vi "rsidr_core_global.vi"() -> ()   [LabVIEW 2015, in "Rohde&Schwarz CMXP NR FR2 Measurement.lvlib"]
doc: "This Global variable contains driver's:\n- Attributes\n- Range Tables\n- Repeated Capabilities"
uses:
  <instrlib>/Rohde&Schwarz CMXP NR FR2 Measurement/Rohde&Schwarz CMXP NR FR2 Measurement.lvlib
panel:
  out "Attributes":T1(array[cluster])=[{"Level"=1, "Class Only"=TRUE, "Identifier"="", "Descriptive Name"="Configuration", "Data Type"=enum."ViInt32", "Command"="", "Access"=enum."Read Only", "Range Table"="", "Read Callback"="", "Write Callback"="", "Range Callback"="", "Check Callback"="", "Rngtable Callback"="", "Coerce Callback"="", "Supported Models"="", "Instrument Options"="", "Check Status Callback"="", "Flags"=0, "Help"="Configures the NR FR 2 measurement subsystem."}, {"Level"=2, "Class Only"=FALSE, "Identifier"="RSCMXPNRFR2M_ATTR_CONNECTOR", "Descriptive Name"="Connector", "Data Type"=enum."ViInt32", "Command"="ROUT:NRMM:MEAS{instance}:SPAT", "Access"=enum."Read/Write", "Range Table"="rsCmxpNrFr2M_rngInputConnector", "Read Callback"="", "Write Callback"="", "Range Callback"="", "Check Callback"="", "Rngtable Callback"="", "Coerce Callback"="", "Supported Models"="", "Instrument Options"="", "Check Status Callback"="", "Flags"=0, "Help"="Selects the input connector for the measured signal.\n\nAvailable Repeated Capabilities:\ninstance: i0, i1, i2, i3, i4, i5, i6, i7, i8, i9, i10, i11, i12, i13, i14, i15, i16, i17, i18, i19, i20, i21, i22, i23, i24, i25, i26, i27, i28, i29, i30, i31, i32\r\n\nRemote-control command(s):\nROUTe:NRMMw:MEAS<i>:SPATh"}, {"Level"=2, "Class Only"=FALSE, "Identifier"="RSCMXPNRFR2M_ATTR_EXTERNAL_ATTENUATION", "Descriptive Name"="External Attenuation", "Data Type"=enum."ViReal64", "Command"="CONF:NRMM:MEAS{instance}:RFS:EATT", "Access"=enum."Read/Write", "Range Table"="rsCmxpNrFr2M_rngExtAtt", "Read Callback"="", "Write Callback"="", "Range Callback"="", "Check Callback"="", "Rngtable Callback"="", "Coerce Callback"="", "Supported Models"="", "Instrument Options"="", "Check Status Callback"="", "Flags"=0, "Help"="Defines an external attenuation (or gain, if the value is negative), to be applied to the input connector.\n\nAvailable Repeated Capabilities:\ninstance: i0, i1, i2, i3, i4, i5, i6, i7, i8, i9, i10, i11, i12, i13, i14, i15, i16, i17, i18, i19, i20, i21, i22, i23, i24, i25, i26, i27, i28, i29, i30, i31, i32\r\n\nRemote-control command(s):\nCONFigure:NRMMw:MEAS<i>:RFSettings:EATTenuation"}, {"Level"=2, "Class Only"=FALSE, "Identifier"="RSCMXPNRFR2M_ATTR_BAND", "Descriptive Name"="Band", "Data Type"=enum."ViInt32", "Command"="CONF:NRMM:MEAS{instance}:BAND", "Access"=enum."Read/Write", "Range Table"="rsCmxpNrFr2M_rngInputSignalFrequencyBand", "Read Callback"="", "Write Callback"="", "Range Callback"="", "Check Callback"="", "Rngtable Callback"="", "Coerce Callback"="", "Supported Models"="", "Instrument Options"="", "Check Status Callback"="", "Flags"=0, "Help"="Selects the frequency band.\n\nAvailable Repeated Capabilities:\ninstance: i0, i1, i2, i3, i4, i5, i6, i7, i8, i9, i10, i11, i12, i13, i14, i15, i16, i17, i18, i19, i20, i21, i22, i23, i24, i25, i26, i27, i28, i29, i30, i31, i32\r\n\nRemote-control command(s):\nCONFigure:NRMMw:MEAS<i>:BAND"}, {"Level"=2, "Class Only"=FALSE, "Identifier"="RSCMXPNRFR2M_ATTR_FREQUENCY", "Descriptive Name"="Frequency", "Data Type"=enum."ViReal64", "Command"="CONF:NRMM:MEAS{instance}:RFS:FREQ", "Access"=enum."Read/Write", "Range Table"="", "Read Callback"="", "Write Callback"="", "Range Callback"="", "Check Callback"="", "Rngtable Callback"="", "Coerce Callback"="", "Supported Models"="", "Instrument Options"="", "Check Status Callback"="", "Flags"=0, "Help"="Selects the center frequency of the measured carrier.\n\nAvailable Repeated Capabilities:\ninstance: i0, i1, i2, i3, i4, i5, i6, i7, i8, i9, i10, i11, i12, i13, i14, i15, i16, i17, i18, i19, i20, i21, i22, i23, i24, i25, i26, i27, i28, i29, i30, i31, i32\r\n\nRemote-control command(s):\nCONFigure:NRMMw:MEAS<i>:RFSettings:FREQuency"}, {"Level"=2, "Class Only"=FALSE, "Identifier"="RSCMXPNRFR2M_ATTR_FREQUENCY_OFFSET", "Descriptive Name"="Frequency Offset", "Data Type"=enum."ViReal64", "Command"="CONF:NRMM:MEAS{instance}:RFS:FOFF", "Access"=enum."Read/Write", "Range Table"="rsCmxpNrFr2M_rngAnalyzerFrequencyOffset", "Read Callback"="", "Write Callback"="", "Range Callback"="", "Check Callback"="", "Rngtable Callback"="", "Coerce Callback"="", "Supported Models"="", "Instrument Options"="", "Check Status Callback"="", "Flags"=0, "Help"="Specifies a positive or negative frequency offset to be added to the carrier center frequency.\n\nAvailable Repeated Capabilities:\ninstance: i0, i1, i2, i3, i4, i5, i6, i7, i8, i9, i10, i11, i12, i13, i14, i15, i16, i17, i18, i19, i20, i21, i22, i23, i24, i25, i26, i27, i28, i29, i30, i31, i32\r\n\nRemote-control command(s):\nCONFigure:NRMMw:MEAS<i>:RFSettings:FOFFset"}, {"Level"=2, "Class Only"=FALSE, "Identifier"="RSCMXPNRFR2M_ATTR_EXPECTED_NOMINAL_POWER", "Descriptive Name"="Expected Nominal Power", "Data Type"=enum."ViReal64", "Command"="CONF:NRMM:MEAS{instance}:RFS:ENP", "Access"=enum."Read/Write", "Range Table"="", "Read Callback"="", "Write Callback"="", "Range Callback"="", "Check Callback"="", "Rngtable Callback"="", "Coerce Callback"="", "Supported Models"="", "Instrument Options"="", "Check Status Callback"="", "Flags"=0, "Help"="Sets the expected nominal power of the measured signal.\n\nAvailable Repeated Capabilities:\ninstance: i0, i1, i2, i3, i4, i5, i6, i7, i8, i9, i10, i11, i12, i13, i14, i15, i16, i17, i18, i19, i20, i21, i22, i23, i24, i25, i26, i27, i28, i29, i30, i31, i32\r\n\nRemote-control command(s):\nCONFigure:NRMMw:MEAS<i>:RFSettings:ENPower"}, {"Level"=2, "Class Only"=FALSE, "Identifier"="RSCMXPNRFR2M_ATTR_USER_MARGIN", "Descriptive Name"="User Margin", "Data Type"=enum."ViReal64", "Command"="CONF:NRMM:MEAS{instance}:RFS:UMAR", "Access"=enum."Read/Write", "Range Table"="", "Read Callback"="", "Write Callback"="", "Range Callback"="", "Check Callback"="", "Rngtable Callback"="", "Coerce Callback"="", "Supported Models"="", "Instrument Options"="", "Check Status Callback"="", "Flags"=0, "Help"="Sets the margin that the measurement adds to the expected nominal power to determine the reference power. The reference power minus the external input attenuation must be within the power range of the selected input connector. Refer to the data sheet.\n\nAvailable Repeated Capabilities:\ninstance: i0, i1, i2, i3, i4, i5, i6, i7, i8, i9, i10, i11, i12, i13, i14, i15, i16, i17, i18, i19, i20, i21, i22, i23, i24, i25, i26, i27, i28, i29, i30, i31, i32\r\n\nRemote-control command(s):\nCONFigure:NRMMw:MEAS<i>:RFSettings:UMARgin"}, {"Level"=2, "Class Only"=FALSE, "Identifier"="RSCMXPNRFR2M_ATTR_MIXER_LEVEL_OFFSET", "Descriptive Name"="Mixer Level Offset", "Data Type"=enum."ViReal64", "Command"="CONF:NRMM:MEAS{instance}:RFS:MLOF", "Access"=enum."Read/Write", "Range Table"="rsCmxpNrFr2M_rngAnalyzerMixerLevelOffset", "Read Callback"="", "Write Callback"="", "Range Callback"="", "Check Callback"="", "Rngtable Callback"="", "Coerce Callback"="", "Supported Models"="", "Instrument Options"="", "Check Status Callback"="", "Flags"=0, "Help"="Varies the input level of the mixer in the analyzer path.\n\nAvailable Repeated Capabilities:\ninstance: i0, i1, i2, i3, i4, i5, i6, i7, i8, i9, i10, i11, i12, i13, i14, i15, i16, i17, i18, i19, i20, i21, i22, i23, i24, i25, i26, i27, i28, i29, i30, i31, i32\r\n\nRemote-control command(s):\nCONFigure:NRMMw:MEAS<i>:RFSettings:MLOFfset"}, {"Level"=2, "Class Only"=FALSE, "Identifier"="RSCMXPNRFR2M_ATTR_RF_UPCONVERSION", "Descriptive Name"="RF Upconversion", "Data Type"=enum."RawString", "Command"="CONF:NRMM:MEAS{instance}:MEV:PCOM", "Access"=enum."Read/Write", "Range Table"="", "Read Callback"="", "Write Callback"="", "Range Callback"="", "Check Callback"="", "Rngtable Callback"="", "Coerce Callback"="", "Supported Models"="", "Instrument Options"="", "Check Status Callback"="", "Flags"=0, "Help"="Specifies the phase compensation applied by the UE during the modulation and upconversion.\n\nSyntax:\nCONFigure:NRMMw:MEAS<i>:MEValuation:PCOMp <PhaseComp>, <UserDefFreq>\n\n<PhaseComp>\nValid Values:\nOFF: no phase compensation\nCAF: phase compensation for carrier frequency\nUDEF: phase compensation for frequency <UserDefFreq>\n \n<UserDefFreq>\n numeric\nFrequency for <PhaseComp> = UDEF\nValid Values: 24.25E+9 Hz  to  52.6E+9 Hz\n\nAvailable Repeated Capabilities:\ninstance: i0, i1, i2, i3, i4, i5, i6, i7, i8, i9, i10, i11, i12, i13, i14, i15, i16, i17, i18, i19, i20, i21, i22, i23, i24, i25, i26, i27, i28, i29, i30, i31, i32\r\n\nRemote-control command(s):\nCONFigure:NRMMw:MEAS<i>:MEValuation:PCOMp"}, {"Level"=2, "Class Only"=TRUE, "Identifier"="", "Descriptive Name"="Signal Settings", "Data Type"=enum."ViInt32", "Command"="", "Access"=enum."Read Only", "Range Table"="", "Read Callback"="", "Write Callback"="", "Range Callback"="", "Check Callback"="", "Rngtable Callback"="", "Coerce Callback"="", "Supported Models"="", "Instrument Options"="", "Check Status Callback"="", "Flags"=0, "Help"="Describe properties of the measured NR signal, that are needed for synchronization and decoding."}, {"Level"=3, "Class Only"=TRUE, "Identifier"="", "Descriptive Name"="TDD UL-DL Configuration", "Data Type"=enum."ViInt32", "Command"="", "Access"=enum."Read Only", "Range Table"="", "Read Callback"="", "Write Callback"="", "Range Callback"="", "Check Callback"="", "Rngtable Callback"="", "Coerce Callback"="", "Supported Models"="", "Instrument Options"="", "Check Status Callback"="", "Flags"=0, "Help"="Settings that configure the UL-DL pattern."}, {"Level"=4, "Class Only"=FALSE, "Identifier"="RSCMXPNRFR2M_ATTR_UL_DL_PERIODICITY", "Descriptive Name"="UL-DL Periodicity", "Data Type"=enum."ViInt32", "Command"="CONF:NRMM:MEAS{instance}:ULDL:PER", "Access"=enum."Read/Write", "Range Table"="rsCmxpNrFr2M_rngPeriodicity", "Read Callback"="", "Write Callback"="", "Range Callback"="", "Check Callback"="", "Rngtable Callback"="", "Coerce Callback"="", "Supported Models"="", "Instrument Options"="", "Check Status Callback"="", "Flags"=0, "Help"="Configures the periodicity of the UL-DL pattern.\n\nAvailable Repeated Capabilities:\ninstance: i0, i1, i2, i3, i4, i5, i6, i7, i8, i9, i10, i11, i12, i13, i14, i15, i16, i17, i18, i19, i20, i21, i22, i23, i24, i25, i26, i27, i28, i29, i30, i31, i32\r\n\nRemote-control command(s):\nCONFigure:NRMMw:MEAS<i>:ULDL:PERiodicity"}, {"Level"=4, "Class Only"=FALSE, "Identifier"="RSCMXPNRFR2M_ATTR_UL_DL_PATTERN", "Descriptive Name"="UL-DL Pattern", "Data Type"=enum."RawString", "Command"="CONF:NRMM:MEAS{instance}:ULDL:PATT", "Access"=enum."Write Only", "Range Table"="", "Read Callback"="", "Write Callback"="", "Range Callback"="", "Check Callback"="", "Rngtable Callback"="", "Coerce Callback"="", "Supported Models"="", "Instrument Options"="", "Check Status Callback"="", "Flags"=0, "Help"="Configures the UL-DL pattern for the <SCSpacing>.\n\nSyntax:\nCONFigure:NRMMw:MEAS<i>:ULDL:PATTern <SCSpacing>, <DLSlots>, <DLSymbols>, <ULSlots>, <ULSymbols>\n\n<SCSpacing>\nSubcarrier spacing for which the other settings apply.\nValid Values:\nS60K\nS120k\n\n<DLSlots>\nnumeric\nSpecifies nrofDownlinkSlots.\nValid Values:  0  to  78 \n\n<DLSymbols>\n numeric\nSpecifies nrofDownlinkSymbols.\nValid Values: 0 to 14 \n\n<ULSlots>\n numeric\nSpecifies nrofUplinkSlots.\nValid Values: 1 to 80 \n\n<ULSymbols>\nnumeric\nSpecifies nrofUplinkSymbols.\nValid Values: 0 to 14\n\nAvailable Repeated Capabilities:\ninstance: i0, i1, i2, i3, i4, i5, i6, i7, i8, i9, i10, i11, i12, i13, i14, i15, i16, i17, i18, i19, i20, i21, i22, i23, i24, i25, i26, i27, i28, i29, i30, i31, i32\r\n\nRemote-control command(s):\nCONFigure:NRMMw:MEAS<i>:ULDL:PATTern"}, {"Level"=4, "Class Only"=FALSE, "Identifier"="RSCMXPNRFR2M_ATTR_HIDDEN_QUERY_UL_DL_PATTERN", "Descriptive Name"="Hidden Query UL-DL Pattern", "Data Type"=enum."RawString", "Command"="CONF:NRMM:MEAS{instance}:ULDL:PATT?", "Access"=enum."Read Only", "Range Table"="", "Read Callback"="", "Write Callback"="", "Range Callback"="", "Check Callback"="", "Rngtable Callback"="", "Coerce Callback"="", "Supported Models"="", "Instrument Options"="", "Check Status Callback"="", "Flags"=8, "Help"="Retrives the UL-DL pattern for the <SCSpacing>.\n\nSyntax:\nCONFigure:NRMMw:MEAS<i>:ULDL:PATTern? <SCSpacing>\n\n<SCSpacing>\nSubcarrier spacing for which the other settings apply.\nValid Values:\nS60K\nS120k\n\nReturned values:\n\n<DLSlots>\nnumeric\nSpecifies nrofDownlinkSlots.\nValid Values:  0  to  78 \n\n<DLSymbols>\n numeric\nSpecifies nrofDownlinkSymbols.\nValid Values: 0 to 14 \n\n<ULSlots>\n numeric\nSpecifies nrofUplinkSlots.\nValid Values: 1 to 80 \n\n<ULSymbols>\nnumeric\nSpecifies nrofUplinkSymbols.\nValid Values: 0 to 14\n\nAvailable Repeated Capabilities:\ninstance: i0, i1, i2, i3, i4, i5, i6, i7, i8, i9, i10, i11, i12, i13, i14, i15, i16, i17, i18, i19, i20, i21, i22, i23, i24, i25, i26, i27, i28, i29, i30, i31, i32\r\n\nRemote-control command(s):\nCONFigure:NRMMw:MEAS<i>:ULDL:PATTern?"}, {"Level"=3, "Class Only"=TRUE, "Identifier"="", "Descriptive Name"="General Carrier Settings", "Data Type"=enum."ViInt32", "Command"="", "Access"=enum."Read Only", "Range Table"="", "Read Callback"="", "Write Callback"="", "Range Callback"="", "Check Callback"="", "Rngtable Callback"="", "Coerce Callback"="", "Supported Models"="", "Instrument Options"="", "Check Status Callback"="", "Flags"=0, "Help"="General carrier settings"}, {"Level"=4, "Class Only"=FALSE, "Identifier"="RSCMXPNRFR2M_ATTR_CHANNEL_BANDWIDTH", "Descriptive Name"="Channel Bandwidth", "Data Type"=enum."ViInt32", "Command"="CONF:NRMM:MEAS{instance}:CC{CC}:CBAN", "Access"=enum."Read/Write", "Range Table"="rsCmxpNrFr2M_rngChannelBandwidth", "Read Callback"="", "Write Callback"="", "Range Callback"="", "Check Callback"="", "Rngtable Callback"="", "Coerce Callback"="", "Supported Models"="", "Instrument Options"="", "Check Status Callback"="", "Flags"=0, "Help"="Specifies the channel bandwidth of carrier <CC>.\n\nAvailable Repeated Capabilities:\ninstance: i0, i1, i2, i3, i4, i5, i6, i7, i8, i9, i10, i11, i12, i13, i14, i15, i16, i17, i18, i19, i20, i21, i22, i23, i24, i25, i26, i27, i28, i29, i30, i31, i32\r\nCC: cc1, cc2\r\n\nRemote-control command(s):\nCONFigure:NRMMw:MEAS<i>[:CC<no>]:CBANdwidth"}, {"Level"=4, "Class Only"=FALSE, "Identifier"="RSCMXPNRFR2M_ATTR_PHYSICAL_CELL_ID", "Descriptive Name"="Physical Cell ID", "Data Type"=enum."ViInt32", "Command"="CONF:NRMM:MEAS{instance}:CC{CC}:PLC", "Access"=enum."Read/Write", "Range Table"="rsCmxpNrFr2M_rngPhysicalCellID", "Read Callback"="", "Write Callback"="", "Range Callback"="", "Check Callback"="", "Rngtable Callback"="", "Coerce Callback"="", "Supported Models"="", "Instrument Options"="", "Check Status Callback"="", "Flags"=0, "Help"="Specifies the physical cell ID of carrier <CC>.\n\nAvailable Repeated Capabilities:\ninstance: i0, i1, i2, i3, i4, i5, i6, i7, i8, i9, i10, i11, i12, i13, i14, i15, i16, i17, i18, i19, i20, i21, i22, i23, i24, i25, i26, i27, i28, i29, i30, i31, i32\r\nCC: cc1, cc2\r\n\nRemote-control command(s):\nCONFigure:NRMMw:MEAS<i>[:CC<no>]:PLCid"}, {"Level"=4, "Class Only"=FALSE, "Identifier"="RSCMXPNRFR2M_ATTR_DMRS_TYPE_A_POSITION", "Descriptive Name"="DMRS Type A Position", "Data Type"=enum."ViInt32", "Command"="CONF:NRMM:MEAS{instance}:CC{CC}:TAP", "Access"=enum."Read/Write", "Range Table"="rsCmxpNrFr2M_rngTypeAPosition", "Read Callback"="", "Write Callback"="", "Range Callback"="", "Check Callback"="", "Rngtable Callback"="", "Coerce Callback"="", "Supported Models"="", "Instrument Options"="", "Check Status Callback"="", "Flags"=0, "Help"="Specifies the 'dmrs-TypeA-Position' for carrier <CC>.\n\nAvailable Repeated Capabilities:\ninstance: i0, i1, i2, i3, i4, i5, i6, i7, i8, i9, i10, i11, i12, i13, i14, i15, i16, i17, i18, i19, i20, i21, i22, i23, i24, i25, i26, i27, i28, i29, i30, i31, i32\r\nCC: cc1, cc2\r\n\nRemote-control command(s):\nCONFigure:NRMMw:MEAS<i>[:CC<no>]:TAPosition"}, {"Level"=4, "Class Only"=FALSE, "Identifier"="RSCMXPNRFR2M_ATTR_SUBCARRIER_SPACING", "Descriptive Name"="Subcarrier Spacing", "Data Type"=enum."ViInt32", "Command"="CONF:NRMM:MEAS{instance}:CCAL:TXBW:SCSP", "Access"=enum."Read/Write", "Range Table"="rsCmxpNrFr2M_rngSubcarrierSpacing", "Read Callback"="", "Write Callback"="", "Range Callback"="", "Check Callback"="", "Rngtable Callback"="", "Coerce Callback"="", "Supported Models"="", "Instrument Options"="", "Check Status Callback"="", "Flags"=0, "Help"="Selects the subcarrier spacing for the measurement, for all carriers.\n\nAvailable Repeated Capabilities:\ninstance: i0, i1, i2, i3, i4, i5, i6, i7, i8, i9, i10, i11, i12, i13, i14, i15, i16, i17, i18, i19, i20, i21, i22, i23, i24, i25, i26, i27, i28, i29, i30, i31, i32\r\n\nRemote-control command(s):\nCONFigure:NRMMw:MEAS<i>:CCALl:TXBWidth:SCSPacing"}, {"Level"=3, "Class Only"=TRUE, "Identifier"="", "Descriptive Name"="Bandwidth Parts", "Data Type"=enum."ViInt32", "Command"="", "Access"=enum."Read Only", "Range Table"="", "Read Callback"="", "Write Callback"="", "Range Callback"="", "Check Callback"="", "Rngtable Callback"="", "Coerce Callback"="", "Supported Models"="", "Instrument Options"="", "Check Status Callback"="", "Flags"=0, "Help"="The settings configure the bandwidth parts of the carrier. In the current software version, you can configure only one bandwidth part."}, {"Level"=4, "Class Only"=FALSE, "Identifier"="RSCMXPNRFR2M_ATTR_BANDWIDTH_PART", "Descriptive Name"="Bandwidth Part", "Data Type"=enum."RawString", "Command"="CONF:NRMM:MEAS{instance}:CC{CC}:BWP", "Access"=enum."Write Only", "Range Table"="", "Read Callback"="", "Write Callback"="", "Range Callback"="", "Check Callback"="", "Rngtable Callback"="", "Coerce Callback"="", "Supported Models"="", "Instrument Options"="", "Check Status Callback"="", "Flags"=0, "Help"="Configures basic properties of the <BWP> on carrier <CC>.\n\nSyntax:\nCONFigure:NRMMw:MEAS<i>[:CC<no>]:BWPart <BWP>, <SCSpacing>, <CyclicPrefix>, <NumberRB>, <StartRB>\n\n<BWP>\nSelects BWP.\nValid Values:\nBWP0\n\n<SCSpacing>\nSubcarrier spacing 60 kHz, 120 kHz.\nValid Values:\nS60K\nS120k\n\n<CyclicPrefix>\nOnly normal CP is supported.\nValid Values:\nNORM\n\n<NumberRB>\nNumber of RBs in the bandwidth part.\ninteger\nValid Values: 11 to 264 \n\n<StartRB>\nIndex of the first RB in the bandwidth part.\ninteger\nValid Values: 0 to 253\n\nAvailable Repeated Capabilities:\ninstance: i0, i1, i2, i3, i4, i5, i6, i7, i8, i9, i10, i11, i12, i13, i14, i15, i16, i17, i18, i19, i20, i21, i22, i23, i24, i25, i26, i27, i28, i29, i30, i31, i32\r\nCC: cc1, cc2\r\n\nRemote-control command(s):\nCONFigure:NRMMw:MEAS<i>[:CC<no>]:BWPart"}, {"Level"=4, "Class Only"=FALSE, "Identifier"="RSCMXPNRFR2M_ATTR_HIDDEN_QUERY_BANDWIDTH_PART", "Descriptive Name"="Hidden Query Bandwidth Part", "Data Type"=enum."RawString", "Command"="CONF:NRMM:MEAS{instance}:CC{CC}:BWP?", "Access"=enum."Read Only", "Range Table"="", "Read Callback"="", "Write Callback"="", "Range Callback"="", "Check Callback"="", "Rngtable Callback"="", "Coerce Callback"="", "Supported Models"="", "Instrument Options"="", "Check Status Callback"="", "Flags"=0, "Help"="Queries basic properties of the <BWP> on carrier <CC>.\n\nSyntax:\nCONFigure:NRMMw:MEAS<i>[:CC<no>]:BWPart? <BWP>\n<SCSpacing>, <CyclicPrefix>, <NumberRB>, <StartRB>\n\nQuery parameter:\n<BWP>\nSelects BWP.\nValid Values:\nBWP0\n\nReturned values:\n<SCSpacing>\nSubcarrier spacing 60 kHz, 120 kHz.\nValid Values:\nS60K\nS120k\n\n<CyclicPrefix>\nOnly normal CP is supported.\nValid Values:\nNORM\n\n<NumberRB>\nNumber of RBs in the bandwidth part.\ninteger\nValid Values: 11 to 264 \n\n<StartRB>\nIndex of the first RB in the bandwidth part.\ninteger\nValid Values: 0 to 253\n\nAvailable Repeated Capabilities:\ninstance: i0, i1, i2, i3, i4, i5, i6, i7, i8, i9, i10, i11, i12, i13, i14, i15, i16, i17, i18, i19, i20, i21, i22, i23, i24, i25, i26, i27, i28, i29, i30, i31, i32\r\nCC: cc1, cc2\r\n\nRemote-control command(s):\nCONFigure:NRMMw:MEAS<i>[:CC<no>]:BWPart?"}, {"Level"=4, "Class Only"=FALSE, "Identifier"="RSCMXPNRFR2M_ATTR_DMRS_FOR_MAPPING_TYPE_A", "Descriptive Name"="DMRS For Mapping Type A", "Data Type"=enum."RawString", "Command"="CONF:NRMM:MEAS{instance}:CC{CC}:BWP:PUSC:DMTA", "Access"=enum."Write Only", "Range Table"="", "Read Callback"="", "Write Callback"="", "Range Callback"="", "Check Callback"="", "Rngtable Callback"="", "Coerce Callback"="", "Supported Models"="", "Instrument Options"="", "Check Status Callback"="", "Flags"=0, "Help"="Configures the DM-RS for mapping type A. The settings apply to the <BWP> on carrier <no>.\n\nSyntax:\nCONFigure:NRMMw:MEAS<i>[:CC<no>]:BWPart:PUSCh:DMTA <BWP>, <ConfigType>, <AddPosition>, <MaxLength>\n\n<BWP>\nSelects BWP.\nValid Values:\nBWP0\n\n<ConfigType>\nDM-RS setting 'dmrs-Type'.\nnumeric\nValid Values: 1 to 2 \n \n<AddPosition>\nDM-RS setting 'dmrs-AdditionalPosition'.\nnumeric\nValid Values: 0 to 3\n\n<MaxLength>\nDM-RS setting 'maxLength'.\nnumeric\nValid Values: 1\n\nAvailable Repeated Capabilities:\ninstance: i0, i1, i2, i3, i4, i5, i6, i7, i8, i9, i10, i11, i12, i13, i14, i15, i16, i17, i18, i19, i20, i21, i22, i23, i24, i25, i26, i27, i28, i29, i30, i31, i32\r\nCC: cc1, cc2\r\n\nRemote-control command(s):\nCONFigure:NRMMw:MEAS<i>[:CC<no>]:BWPart:PUSCh:DMTA"}, {"Level"=4, "Class Only"=FALSE, "Identifier"="RSCMXPNRFR2M_ATTR_DMRS_FOR_MAPPING_TYPE_B", "Descriptive Name"="DMRS For Mapping Type B", "Data Type"=enum."RawString", "Command"="CONF:NRMM:MEAS{instance}:CC{CC}:BWP:PUSC:DMTB", "Access"=enum."Write Only", "Range Table"="", "Read Callback"="", "Write Callback"="", "Range Callback"="", "Check Callback"="", "Rngtable Callback"="", "Coerce Callback"="", "Supported Models"="", "Instrument Options"="", "Check Status Callback"="", "Flags"=0, "Help"="Configures the DM-RS for mapping type A. The settings apply to the <BWP> on carrier <no>.\n\nSyntax:\nCONFigure:NRMMw:MEAS<i>[:CC<no>]:BWPart:PUSCh:DMTA <BWP>, <ConfigType>, <AddPosition>, <MaxLength>\n\n<BWP>\nSelects BWP.\nValid Values:\nBWP0\n\n<ConfigType>\nDM-RS setting 'dmrs-Type'.\nnumeric\nValid Values: 1 to 2 \n \n<AddPosition>\nDM-RS setting 'dmrs-AdditionalPosition'.\nnumeric\nValid Values: 0 to 3\n\n<MaxLength>\nDM-RS setting 'maxLength'.\nnumeric\nValid Values: 1\n\nAvailable Repeated Capabilities:\ninstance: i0, i1, i2, i3, i4, i5, i6, i7, i8, i9, i10, i11, i12, i13, i14, i15, i16, i17, i18, i19, i20, i21, i22, i23, i24, i25, i26, i27, i28, i29, i30, i31, i32\r\nCC: cc1, cc2\r\n\nRemote-control command(s):\nCONFigure:NRMMw:MEAS<i>[:CC<no>]:BWPart:PUSCh:DMTB"}, {"Level"=4, "Class Only"=FALSE, "Identifier"="RSCMXPNRFR2M_ATTR_HIDDEN_QUERY_DMRS_FOR_MAPPING_TYPE_A", "Descriptive Name"="Hidden Query DMRS For Mapping Type A", "Data Type"=enum."RawString", "Command"="CONF:NRMM:MEAS{instance}:CC{CC}:BWP:PUSC:DMTA?", "Access"=enum."Read Only", "Range Table"="", "Read Callback"="", "Write Callback"="", "Range Callback"="", "Check Callback"="", "Rngtable Callback"="", "Coerce Callback"="", "Supported Models"="", "Instrument Options"="", "Check Status Callback"="", "Flags"=8, "Help"="Configures the DM-RS for mapping type A. The settings apply to the <BWP> on carrier <no>.\n\nSyntax:\nCONFigure:NRMMw:MEAS<i>[:CC<no>]:BWPart:PUSCh:DMTA <BWP>\n<ConfigType>, <AddPosition>, <MaxLength>\n\nQuery parameters:\n<BWP>\nSelects BWP.\nValid Values:\nBWP0\n\nReturned values:\n<ConfigType>\nDM-RS setting 'dmrs-Type'.\nnumeric\nValid Values: 1 to 2 \n \n<AddPosition>\nDM-RS setting 'dmrs-AdditionalPosition'.\nnumeric\nValid Values: 0 to 3\n\n<MaxLength>\nDM-RS setting 'maxLength'.\nnumeric\nValid Values: 1\n\nAvailable Repeated Capabilities:\ninstance: i0, i1, i2, i3, i4, i5, i6, i7, i8, i9, i10, i11, i12, i13, i14, i15, i16, i17, i18, i19, i20, i21, i22, i23, i24, i25, i26, i27, i28, i29, i30, i31, i32\r\nCC: cc1, cc2\r\n\nRemote-control command(s):\nCONFigure:NRMMw:MEAS<i>[:CC<no>]:BWPart:PUSCh:DMTA?"}, {"Level"=4, "Class Only"=FALSE, "Identifier"="RSCMXPNRFR2M_ATTR_HIDDEN_QUERY_DMRS_FOR_MAPPING_TYPE_B", "Descriptive Name"="Hidden Query DMRS For Mapping Type B", "Data Type"=enum."RawString", "Command"="CONF:NRMM:MEAS{instance}:CC{CC}:BWP:PUSC:DMTB?", "Access"=enum."Read Only", "Range Table"="", "Read Callback"="", "Write Callback"="", "Range Callback"="", "Check Callback"="", "Rngtable Callback"="", "Coerce Callback"="", "Supported Models"="", "Instrument Options"="", "Check Status Callback"="", "Flags"=0, "Help"="Configures the DM-RS for mapping type A. The settings apply to the <BWP> on carrier <no>.\n\nSyntax:\nCONFigure:NRMMw:MEAS<i>[:CC<no>]:BWPart:PUSCh:DMTA <BWP>\n<ConfigType>, <AddPosition>, <MaxLength>\n\nQuery parameters:\n<BWP>\nSelects BWP.\nValid Values:\nBWP0\n\nReturned parameters:\n<ConfigType>\nDM-RS setting 'dmrs-Type'.\nnumeric\nValid Values: 1 to 2 \n \n<AddPosition>\nDM-RS setting 'dmrs-AdditionalPosition'.\nnumeric\nValid Values: 0 to 3\n\n<MaxLength>\nDM-RS setting 'maxLength'.\nnumeric\nValid Values: 1\n\nAvailable Repeated Capabilities:\ninstance: i0, i1, i2, i3, i4, i5, i6, i7, i8, i9, i10, i11, i12, i13, i14, i15, i16, i17, i18, i19, i20, i21, i22, i23, i24, i25, i26, i27, i28, i29, i30, i31, i32\r\nCC: cc1, cc2\r\n\nRemote-control command(s):\nCONFigure:NRMMw:MEAS<i>[:CC<no>]:BWPart:PUSCh:DMTB?"}, {"Level"=4, "Class Only"=FALSE, "Identifier"="RSCMXPNRFR2M_ATTR_TRANSFORM_PRECODING", "Descriptive Name"="Transform Precoding", "Data Type"=enum."RawString", "Command"="CONF:NRMM:MEAS{instance}:CC{CC}:BWP:PUSC:DFTP", "Access"=enum."Write Only", "Range Table"="", "Read Callback"="", "Write Callback"="", "Range Callback"="", "Check Callback"="", "Rngtable Callback"="", "Coerce Callback"="", "Supported Models"="", "Instrument Options"="", "Check Status Callback"="", "Flags"=0, "Help"="Specifies whether the <BWP> on carrier <no> uses a transform precoding function.\n\nSyntax:\n<BWP>\nSelects BWP.\nValid Values:\nBWP0\n\n<Enable>\nValid Values:\nOFF - No transform precoding\nON - With transform precoding\n\nAvailable Repeated Capabilities:\ninstance: i0, i1, i2, i3, i4, i5, i6, i7, i8, i9, i10, i11, i12, i13, i14, i15, i16, i17, i18, i19, i20, i21, i22, i23, i24, i25, i26, i27, i28, i29, i30, i31, i32\r\nCC: cc1, cc2\r\n\nRemote-control command(s):\nCONFigure:NRMMw:MEAS<i>[:CC<no>]:BWPart:PUSCh:DFTPrecoding"}, {"Level"=4, "Class Only"=FALSE, "Identifier"="RSCMXPNRFR2M_ATTR_HIDDEN_QUERY_TRANSFORM_PRECODING", "Descriptive Name"="Hidden Query Transform Precoding", "Data Type"=enum."ViBoolean", "Command"="CONF:NRMM:MEAS{instance}:CC{CC}:BWP:PUSC:DFTP?", "Access"=enum."Read Only", "Range Table"="", "Read Callback"="", "Write Callback"="", "Range Callback"="", "Check Callback"="", "Rngtable Callback"="", "Coerce Callback"="", "Supported Models"="", "Instrument Options"="", "Check Status Callback"="", "Flags"=8, "Help"="Query whether the <BWP> on carrier <no> uses a transform precoding function.\n\nSyntax:\n<BWP>\nSelects BWP.\nValid Values:\nBWP0\n\nValid Values:\nOFF - No transform precoding\nON - With transform precoding\n\nAvailable Repeated Capabilities:\ninstance: i0, i1, i2, i3, i4, i5, i6, i7, i8, i9, i10, i11, i12, i13, i14, i15, i16, i17, i18, i19, i20, i21, i22, i23, i24, i25, i26, i27, i28, i29, i30, i31, i32\r\nCC: cc1, cc2\r\n\nRemote-control command(s):\nCONFigure:NRMMw:MEAS<i>[:CC<no>]:BWPart:PUSCh:DFTPrecoding?"}, {"Level"=3, "Class Only"=TRUE, "Identifier"="", "Descriptive Name"="Scheduled Slot Allocation", "Data Type"=enum."ViInt32", "Command"="", "Access"=enum."Read Only", "Range Table"="", "Read Callback"="", "Write Callback"="", "Range Callback"="", "Check Callback"="", "Rngtable Callback"="", "Coerce Callback"="", "Supported Models"="", "Instrument Options"="", "Check Status Callback"="", "Flags"=0, "Help"="Scheduled Slot Allocation"}, {"Level"=4, "Class Only"=FALSE, "Identifier"="RSCMXPNRFR2M_ATTR_COMMON_PUSCH_ALLOCATION", "Descriptive Name"="Common PUSCH Allocation", "Data Type"=enum."RawString", "Command"="CONF:NRMM:MEAS{instance}:CC{CC}:ALL{Allocation}:PUSC", "Access"=enum."Read/Write", "Range Table"="", "Read Callback"="", "Write Callback"="", "Range Callback"="", "Check Callback"="", "Rngtable Callback"="", "Coerce Callback"="", "Supported Models"="", "Instrument Options"="", "Check Status Callback"="", "Flags"=0, "Help"="Specifies settings related to the PUSCH allocation, for carrier <no>, allocation <a>.\n\nSyntax:\nCONFigure:NRMMw:MEAS<i>[:CC<no>]:ALLocation<a>:PUSCh <MappingType>, <NoSymbols>, <StartSymbol>, <NoRBs>, <StartRB>, <ModScheme>\n\n<MappingType>\nPUSCH mapping type\nValid Values:\nA\nB\n  \n<NoSymbols>\nNumber of allocated OFDM symbols in each uplink slot.\nnumeric\nValid Values: 4 to 14 \n \n<StartSymbol>\nIndex of the first allocated symbol in each uplink slot.\nFor mapping type A, only 0 is allowed.\nnumeric\nValid Values: 0 to 10\n\n<NoRBs>\nNumber of allocated UL RBs.\nnumeric\nValid Values: 1 to 264 \n\n<StartRB>\nIndex of the first allocated RB.\nnumeric\nValid Values: 0 to 263 \n\n<ModScheme>\nModulation scheme\nValid Values:\nPHBPsk - Pi/2-BPSK\nQPSK - QPSK\nQ16 - 16-QAM\nQ64 - 64-QAM\nQ256 - 256-QAM\n\nAvailable Repeated Capabilities:\ninstance: i0, i1, i2, i3, i4, i5, i6, i7, i8, i9, i10, i11, i12, i13, i14, i15, i16, i17, i18, i19, i20, i21, i22, i23, i24, i25, i26, i27, i28, i29, i30, i31, i32\r\nCC: cc1, cc2\r\nAllocation: alloc1\r\n\nRemote-control command(s):\nCONFigure:NRMMw:MEAS<i>[:CC<no>]:ALLocation<a>:PUSCh"}, {"Level"=4, "Class Only"=FALSE, "Identifier"="RSCMXPNRFR2M_ATTR_ADDITIONAL_PUSCH_ALLOCATION", "Descriptive Name"="Additional PUSCH Allocation", "Data Type"=enum."RawString", "Command"="CONF:NRMM:MEAS{instance}:CC{CC}:ALL{Allocation}:PUSC:ADD", "Access"=enum."Read/Write", "Range Table"="", "Read Callback"="", "Write Callback"="", "Range Callback"="", "Check Callback"="", "Rngtable Callback"="", "Coerce Callback"="", "Supported Models"="", "Instrument Options"="", "Check Status Callback"="", "Flags"=0, "Help"="Configures special PUSCH settings, for carrier <no>, allocation <a>.\n\nSyntax:\nCONFigure:NRMMw:MEAS<i>[:CC<no>]:ALLocation<a>:PUSCh:ADDitional <DMRSLength>,<CDMGroups>,DMRSPower>,<AntennaPort>\n\n<DMRSLength>\nLength of the DM-RS in symbols. The maximum value is limited by the 'maxLength' setting for the bandwidth part.\nnumeric\nValid Values: 1\n\n<CDMGroups>\nNumber of DM-RS CDM groups without data.\nnumeric\nValid Values: 1 to 3\n\n<DMRSPower>\nPower of DM-RS relative to the PUSCH power.\nnumeric\nValid Values: -10 dB to 10 dB\n\n<AntennaPort>\nAntenna port of the DM-RS.\nnumeric\nValid Values: 0 to 1\n\nAvailable Repeated Capabilities:\ninstance: i0, i1, i2, i3, i4, i5, i6, i7, i8, i9, i10, i11, i12, i13, i14, i15, i16, i17, i18, i19, i20, i21, i22, i23, i24, i25, i26, i27, i28, i29, i30, i31, i32\r\nCC: cc1, cc2\r\nAllocation: alloc1\r\n\nRemote-control command(s):\nCONFigure:NRMMw:MEAS<i>[:CC<no>]:ALLocation<a>:PUSCh:ADDitional"}, {"Level"=4, "Class Only"=FALSE, "Identifier"="RSCMXPNRFR2M_ATTR_DRMS_SEQUENCE_GENERATION", "Descriptive Name"="DR-MS Sequence Generation", "Data Type"=enum."RawString", "Command"="CONF:NRMM:MEAS{instance}:CC{CC}:ALL{Allocation}:PUSC:SGEN", "Access"=enum."Read/Write", "Range Table"="", "Read Callback"="", "Write Callback"="", "Range Callback"="", "Check Callback"="", "Rngtable Callback"="", "Coerce Callback"="", "Supported Models"="", "Instrument Options"="", "Check Status Callback"="", "Flags"=0, "Help"="Configures the initialization of the DM-RS sequence generation, for carrier <no>, allocation <a>.\n\nSyntax:\nCONFigure:NRMMw:MEAS<i>[:CC<no>]:ALLocation<a>:PUSCh:SGENeration <Initialization>, <DMRSID>, <N_SCID>\n\n<Initialization>\nUsed ID\nValid Values:\nCID - cell ID used\nDMRSid - DMRS ID used\n \n<DMRSID>\nID for <Initialization> = DMRSid.\nnumeric\nValid Values: 0 to 65535 \n\n<N_SCID>\nParameter nSCID.\nnumeric\nValid Values: 0 to 1\n\nAvailable Repeated Capabilities:\ninstance: i0, i1, i2, i3, i4, i5, i6, i7, i8, i9, i10, i11, i12, i13, i14, i15, i16, i17, i18, i19, i20, i21, i22, i23, i24, i25, i26, i27, i28, i29, i30, i31, i32\r\nCC: cc1, cc2\r\nAllocation: alloc1\r\n\nRemote-control command(s):\nCONFigure:NRMMw:MEAS<i>[:CC<no>]:ALLocation<a>:PUSCh:SGENeration"}, {"Level"=1, "Class Only"=TRUE, "Identifier"="", "Descriptive Name"="Multi Evaluation Measurement", "Data Type"=enum."ViInt32", "Command"="", "Access"=enum."Read Only", "Range Table"="", "Read Callback"="", "Write Callback"="", "Range Callback"="", "Check Callback"="", "Rngtable Callback"="", "Coerce Callback"="", "Supported Models"="", "Instrument Options"="", "Check Status Callback"="", "Flags"=0, "Help"="WLAN \"Multi Evaluation\" measurement"}, {"Level"=2, "Class Only"=TRUE, "Identifier"="", "Descriptive Name"="Control and States", "Data Type"=enum."ViInt32", "Command"="", "Access"=enum."Read Only", "Range Table"="", "Read Callback"="", "Write Callback"="", "Range Callback"="", "Check Callback"="", "Rngtable Callback"="", "Coerce Callback"="", "Supported Models"="", "Instrument Options"="", "Check Status Callback"="", "Flags"=0, "Help"="Measurement control and states."}, {"Level"=3, "Class Only"=FALSE, "Identifier"="RSCMXPNRFR2M_ATTR_MULTI_EVAL_MEASUREMENT_INIT", "Descriptive Name"="Multi Eval Measurement Init", "Data Type"=enum."None", "Command"="INIT:NRMM:MEAS{instance}:MEV", "Access"=enum."Write Only", "Range Table"="", "Read Callback"="", "Write Callback"="", "Range Callback"="", "Check Callback"="", "Rngtable Callback"="", "Coerce Callback"="", "Supported Models"="", "Instrument Options"="", "Check Status Callback"="", "Flags"=1, "Help"="Starts or restarts the measurement; the measurement enters the 'RUN' state.\n\nAvailable Repeated Capabilities:\ninstance: i0, i1, i2, i3, i4, i5, i6, i7, i8, i9, i10, i11, i12, i13, i14, i15, i16, i17, i18, i19, i20, i21, i22, i23, i24, i25, i26, i27, i28, i29, i30, i31, i32\r\n\nRemote-control command(s):\nINITiate:NRMMw:MEAS<i>:MEValuation"}, {"Level"=3, "Class Only"=FALSE, "Identifier"="RSCMXPNRFR2M_ATTR_MULTI_EVAL_MEASUREMENT_ABORT", "Descriptive Name"="Multi Eval Measurement Abort", "Data Type"=enum."None", "Command"="ABOR:NRMM:MEAS{instance}:MEV", "Access"=enum."Write Only", "Range Table"="", "Read Callback"="", "Write Callback"="", "Range Callback"="", "Check Callback"="", "Rngtable Callback"="", "Coerce Callback"="", "Supported Models"="", "Instrument Options"="", "Check Status Callback"="", "Flags"=0, "Help"="Causes a running measurement to stop immediately; the measurement enters the 'OFF' state. All measurement values are set to NAV. Allocated resources are released.\n\nAvailable Repeated Capabilities:\ninstance: i0, i1, i2, i3, i4, i5, i6, i7, i8, i9, i10, i11, i12, i13, i14, i15, i16, i17, i18, i19, i20, i21, i22, i23, i24, i25, i26, i27, i28, i29, i30, i31, i32\r\n\nRemote-control command(s):\nABORt:NRMMw:MEAS<i>:MEValuation"}, {"Level"=3, "Class Only"=FALSE, "Identifier"="RSCMXPNRFR2M_ATTR_MULTI_EVAL_MEASUREMENT_STOP", "Descriptive Name"="Multi Eval Measurement Stop", "Data Type"=enum."None", "Command"="STOP:NRMM:MEAS{instance}:MEV", "Access"=enum."Write Only", "Range Table"="", "Read Callback"="", "Write Callback"="", "Range Callback"="", "Check Callback"="", "Rngtable Callback"="", "Coerce Callback"="", "Supported Models"="", "Instrument Options"="", "Check Status Callback"="", "Flags"=0, "Help"="Causes a running measurement to stop immediately; the measurement enters the 'RDY' state. Measurement results are kept. The resources remain allocated to the measurement.\n\nAvailable Repeated Capabilities:\ninstance: i0, i1, i2, i3, i4, i5, i6, i7, i8, i9, i10, i11, i12, i13, i14, i15, i16, i17, i18, i19, i20, i21, i22, i23, i24, i25, i26, i27, i28, i29, i30, i31, i32\r\n\nRemote-control command(s):\nSTOP:NRMMw:MEAS<i>:MEValuation"}, {"Level"=3, "Class Only"=FALSE, "Identifier"="RSCMXPNRFR2M_ATTR_MULTI_EVAL_MEASUREMENT_MEASUREMENT_STATE", "Descriptive Name"="Multi Eval Measurement Measurement State", "Data Type"=enum."RawString", "Command"="FETC:NRMM:MEAS{instance}:MEV:STAT:ALL?", "Access"=enum."Read Only", "Range Table"="", "Read Callback"="", "Write Callback"="", "Range Callback"="", "Check Callback"="", "Rngtable Callback"="", "Coerce Callback"="", "Supported Models"="", "Instrument Options"="", "Check Status Callback"="", "Flags"=0, "Help"="Queries the main measurement state and the measurement substates. Both measurement substates are relevant for running measurements only. Use FETCh:...:STATe? to query the main measurement state only. Use INITiate..., STOP..., ABORt... to change the measurement state.\n\nAvailable Repeated Capabilities:\ninstance: i0, i1, i2, i3, i4, i5, i6, i7, i8, i9, i10, i11, i12, i13, i14, i15, i16, i17, i18, i19, i20, i21, i22, i23, i24, i25, i26, i27, i28, i29, i30, i31, i32\r\n\nRemote-control command(s):\nFETCh:NRMMw:MEAS<i>:MEValuation:STATe:ALL?"}, {"Level"=2, "Class Only"=TRUE, "Identifier"="", "Descriptive Name"="Configuration", "Data Type"=enum."ViInt32", "Command"="", "Access"=enum."Read Only", "Range Table"="", "Read Callback"="", "Write Callback"="", "Range Callback"="", "Check Callback"="", "Rngtable Callback"="", "Coerce Callback"="", "Supported Models"="", "Instrument Options"="", "Check Status Callback"="", "Flags"=0, "Help"="Multi Evaluation measurement configuration attributes."}, {"Level"=3, "Class Only"=TRUE, "Identifier"="", "Descriptive Name"="Control", "Data Type"=enum."ViInt32", "Command"="", "Access"=enum."Read Only", "Range Table"="", "Read Callback"="", "Write Callback"="", "Range Callback"="", "Check Callback"="", "Rngtable Callback"="", "Coerce Callback"="", "Supported Models"="", "Instrument Options"="", "Check Status Callback"="", "Flags"=0, "Help"="General measurement control settings"}, {"Level"=4, "Class Only"=FALSE, "Identifier"="RSCMXPNRFR2M_ATTR_MULTI_EVAL_MEASUREMENT_REPETITION", "Descriptive Name"="Multi Eval Measurement Repetition", "Data Type"=enum."ViInt32", "Command"="CONF:NRMM:MEAS{instance}:MEV:REP", "Access"=enum."Read/Write", "Range Table"="rsCmxpNrFr2M_rngRepMode", "Read Callback"="", "Write Callback"="", "Range Callback"="", "Check Callback"="", "Rngtable Callback"="", "Coerce Callback"="", "Supported Models"="", "Instrument Options"="", "Check Status Callback"="", "Flags"=0, "Help"="Specifies the repetition mode of the measurement. The repetition mode specifies whether the measurement is stopped after a single shot or repeated continuously. Use CONFigure:..:MEAS<i>:...:SCOunt to determine the number of measurement intervals per single shot.\n\nAvailable Repeated Capabilities:\ninstance: i0, i1, i2, i3, i4, i5, i6, i7, i8, i9, i10, i11, i12, i13, i14, i15, i16, i17, i18, i19, i20, i21, i22, i23, i24, i25, i26, i27, i28, i29, i30, i31, i32\r\n\nRemote-control command(s):\nCONFigure:NRMMw:MEAS<i>:MEValuation:REPetition"}, {"Level"=4, "Class Only"=FALSE, "Identifier"="RSCMXPNRFR2M_ATTR_MULTI_EVAL_MEASUREMENT_STOP_CONDITION", "Descriptive Name"="Multi Eval Measurement Stop Condition", "Data Type"=enum."ViInt32", "Command"="CONF:NRMM:MEAS{instance}:MEV:SCON", "Access"=enum."Read/Write", "Range Table"="rsCmxpNrFr2M_rngStopCondition", "Read Callback"="", "Write Callback"="", "Range Callback"="", "Check Callback"="", "Rngtable Callback"="", "Coerce Callback"="", "Supported Models"="", "Instrument Options"="", "Check Status Callback"="", "Flags"=0, "Help"="Qualifies whether the measurement is stopped after a failed limit check or continued. SLFail means that the measurement is stopped and reaches the RDY state when one of the results exceeds the limits.\n\nAvailable Repeated Capabilities:\ninstance: i0, i1, i2, i3, i4, i5, i6, i7, i8, i9, i10, i11, i12, i13, i14, i15, i16, i17, i18, i19, i20, i21, i22, i23, i24, i25, i26, i27, i28, i29, i30, i31, i32\r\n\nRemote-control command(s):\nCONFigure:NRMMw:MEAS<i>:MEValuation:SCONdition"}, {"Level"=4, "Class Only"=FALSE, "Identifier"="RSCMXPNRFR2M_ATTR_DISABLE_MULTI_EVAL_MEASUREMENT_MODE", "Descriptive Name"="Disable Multi Eval Measurement Mode", "Data Type"=enum."None", "Command"="CONF:NRMM:MEAS{instance}:MEV:MMOD NORM", "Access"=enum."Write Only", "Range Table"="", "Read Callback"="", "Write Callback"="", "Range Callback"="", "Check Callback"="", "Rngtable 
